vi "INSPECT_Wait for Start Pos Helper.vi"(8 "error in (no error)":errorcluster, 10 "Inspect Helper Loop Data":T1={"Inspect State"=enum."Init", "Timeout"=0, "Loop Count"=0, "Start Sample No."=0, "Inspect Status "={"Ready"=FALSE, "Inspecting"=FALSE, "Cancel"=FALSE}, "Encoder Count"=0, "PosToStartScan"=50800, "ScanLength"=50800, "MaxSamples"=50800, "PosToEndScan"=0, "Host SampleData"=refnum, "data value reference"=refnum, "Block Cnt notifier out"=refnum, "STATUS"={"Initialized"=FALSE, "Connected"=FALSE, "Ready"=FALSE, "Inspecting"=FALSE, "Position"=0.0, "Status"=0, "Error"=FALSE, "Code"=0, "MC SM State"=0, "M_Ctrl"=0}, "EventLog"=refnum}, 11 "Message Queue in":refnum<class "Delacor_lib_QMH_Message Queue.lvclass">) -> (0 "error out":errorcluster, 2 "Inspect Helper Loop Data out":T1={"Inspect State"=enum."Init", "Timeout"=0, "Loop Count"=0, "Start Sample No."=0, "Inspect Status "={"Ready"=FALSE, "Inspecting"=FALSE, "Cancel"=FALSE}, "Encoder Count"=0, "PosToStartScan"=50800, "ScanLength"=50800, "MaxSamples"=50800, "PosToEndScan"=0, "Host SampleData"=refnum, "data value reference"=refnum, "Block Cnt notifier out"=refnum, "STATUS"={"Initialized"=FALSE, "Connected"=FALSE, "Ready"=FALSE, "Inspecting"=FALSE, "Position"=0.0, "Status"=0, "Error"=FALSE, "Code"=0, "MC SM State"=0, "M_Ctrl"=0}, "EventLog"=refnum})   [LabVIEW 2015, in "Tool Module.lvlib"]
uses:
  Tool Module.lvlib
  _Inspect Helper Loop Data Cluster--typedef.ctl
  Event Logger Library/Event Log/EventLog.lvclass
  _Inspect SM Enum--typedef.ctl
  _Inspect Status Update Cluster--typedef.ctl
  _Sample Data Rtn Cluster--typedef.ctl
  _STATUS Typedef--cluster.ctl
  <vilib>/Delacor/Delacor QMH/Libraries/Message Queue_class/Delacor_lib_QMH_Message Queue.lvclass
  <vilib>/Delacor/Delacor QMH/Libraries/Message Queue_class/Delacor_lib_QMH_Message Queue.lvclass/Delacor_lib_QMH_Message Queue.ctl
  <vilib>/Delacor/Delacor QMH/Libraries/Message Queue_class/Delacor_lib_QMH_Enqueue Message (Single).vi
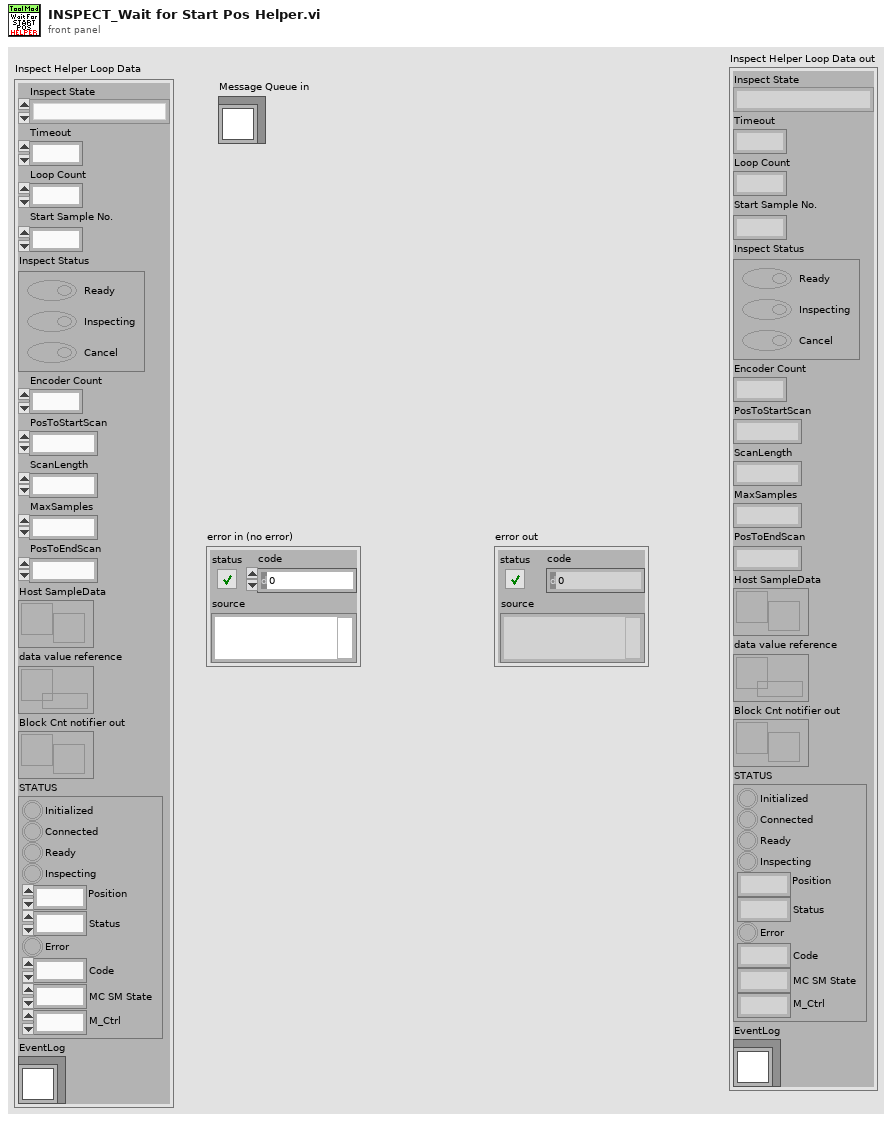
[diagram p1: front panel]
types:
  T1 = typedef "Tool Module.lvlib/_Inspect Helper Loop Data Cluster--typedef.ctl" = cluster{"Inspect State":T2, "Timeout":i32, "Loop Count":i32, "Start Sample No.":u32, "Inspect Status ":T3, "Encoder Count":i32, "PosToStartScan":i32, "ScanLength":i32, "MaxSamples":i32, "PosToEndScan":i32, "Host SampleData":refnum<notifier>, "data value reference":refnum<data-value>, "Block Cnt notifier out":refnum<notifier>, "STATUS":T4, "EventLog":refnum<class "EventLog.lvclass">}
  T2 = typedef "Tool Module.lvlib/_Inspect SM Enum--typedef.ctl" = enum16{"Init", "Set Motion Speed", "Move To Scan Start", "Wait for Motion Out", "Wait for Start Pos", "Delay before Motion IN", "Start Inspecting", "Wait for Motion IN", "Wait for Inspect Range", "Delay before Inspecting", "Inspecting", "Stop Inspecting"}
  T3 = typedef "Tool Module.lvlib/_Inspect Status Update Cluster--typedef.ctl" = cluster{"Ready":bool, "Inspecting":bool, "Cancel":bool}
  T4 = typedef "Tool Module.lvlib/_STATUS Typedef--cluster.ctl" = cluster{"Initialized":bool, "Connected":bool, "Ready":bool, "Inspecting":bool, "Position":dbl, "Status":u16, "Error":bool, "Code":i32, "MC SM State":u16, "M_Ctrl":u16}
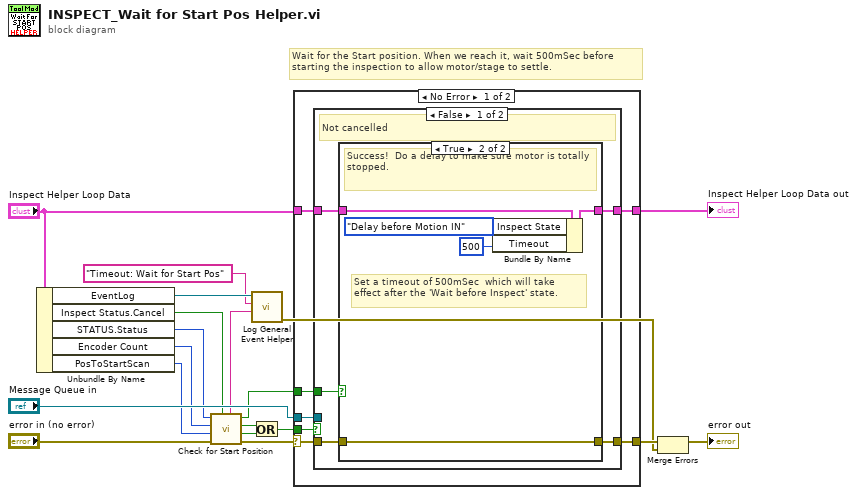
[diagram p0: block diagram]
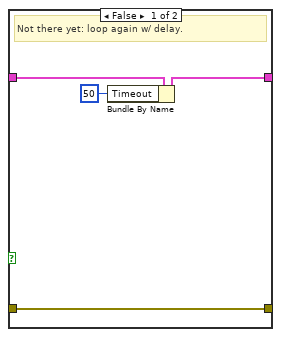
[diagram p2: hidden frame]
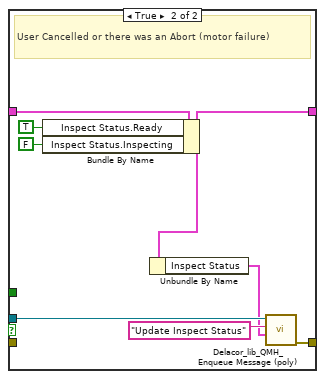
[diagram p3: hidden frame]
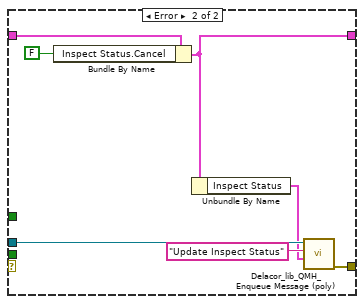
[diagram p4: hidden frame]
diagram:
  # "Wait for the Start position. When we reach it, wait 500mSec before starting the inspection to allow motor/stage to settle."
  n1 = Unbundle By Name("Inspect Helper Loop Data") -> ("EventLog"=w5:refnum<class "EventLog.lvclass">, "Inspect Status.Cancel"=w17:bool, "STATUS.Status"=w16:u16, "Encoder Count"=w15:i32, "PosToStartScan"=w14:i32)
  n2 = call "Check for Start Position.vi"("Cancel Inspect"=w17, "error in (no error)"="error in (no error)", "Target Encdr Pos."=w14, "Cur Encoder Value"=w15, "Status Byte"=w16) -> ("error out"=w19:errorcluster, "Aborted"=w11:bool, "Cancelled"=w10:bool, "Success"=w8:bool, "Log String out"=w4:string)  [unwired: 2 in]
  n3 = call "Log General Event Helper.vi"("Payload"=w4, "State Info"="Timeout: Wait for Start Pos", "EventLog in"=w5) -> ("error out"=w1:errorcluster)  [unwired: 7 in, 1 out]
  n4 = Or(x=w10, y=w11) -> (x .or. y?=w9:bool)
  n5 = case shown="No Error" w19 {
    selector: w19 -> [w20 _]
    tunnel: [w26 w53] -> w7
    tunnel: "Message Queue in" -> [w25 w52]
    tunnel: "Inspect Helper Loop Data" -> [w24 w55]
    tunnel: [w23 w50] -> w6
    tunnel: w9 -> [w22 _]
    tunnel: w8 -> [w21 _]
    frame No Error {
      n6 = case shown="False" w22 {
        tunnel: [w27 w48] -> w26
        tunnel: w25 -> [_ w47]
        tunnel: w24 -> [w29 w45]
        tunnel: [w28 w44] -> w23
        tunnel: w21 -> [w31 _]
        tunnel: w20 -> [w30 _]
        frame False {
          # "Not cancelled"
          n7 = case shown="True" w31 {
            tunnel: w30 -> [w32 w36]
            tunnel: w29 -> [w35 w40]
            tunnel: [w34 w39] -> w28
            tunnel: [w32 w36] -> w27
            frame False {
              # "Not there yet: loop again w/ delay."
              n8 = Bundle By Name(cluster=w35, "Timeout"=50) -> (w34:T1)
            }
            frame True {
              # "Set a timeout of 500mSec  which will take effect after the 'Wait before Inspect' state."
              # "Success!  Do a delay to make sure motor is totally stopped."
              n9 = Bundle By Name(cluster=w40, "Inspect State"=_Inspect_SM_Enum--typedef."Delay before Motion IN", "Timeout"=500) -> (w39:T1)
            }
          }
        }
        frame True {
          # "User Cancelled or there was an Abort (motor failure)"
          n10 = Bundle By Name(cluster=w45, "Inspect Status.Ready"=TRUE ("Inspect Status .Ready"), "Inspect Status.Inspecting"=FALSE ("Inspect Status .Inspecting")) -> (w44:T1)
          n11 = Unbundle By Name(w44) -> ("Inspect Status"=w41:T3)
          n12 = call-poly <vilib>:"Delacor_lib_QMH_Enqueue Message (poly).vi"("Message Data"=w41, "Message"="Update Inspect Status", "Message Queue in"=w47) -> ("error out"=w48:errorcluster)  [unwired: 7 in, 1 out]
        }
      }
    }
    frame Error {
      n13 = Bundle By Name(cluster=w55, "Inspect Status.Cancel"=FALSE ("Inspect Status .Cancel")) -> (w50:T1)
      n14 = Unbundle By Name(w50) -> ("Inspect Status"=w49:T3)
      n15 = call-poly <vilib>:"Delacor_lib_QMH_Enqueue Message (poly).vi"("Message Data"=w49, "Message"="Update Inspect Status", "Message Queue in"=w52) -> ("error out"=w53:errorcluster)  [unwired: 7 in, 1 out]
    }
  }
  "Inspect Helper Loop Data out" <- w6
  n16 = Merge Errors(w7, w1) -> (→"error out":errorcluster)
